vi "writeSerialCommunicator.vi"(8 "error in (no error)":errorcluster, 10 "serialCommunicator":refnum<class "SerialCommunicator.lvclass">, 11 "TEI9150 in":refnum<class "Tovey9150.lvclass">) -> (0 "error out":errorcluster, 3 "TEI9150 out":refnum<class "Tovey9150.lvclass">)   [LabVIEW 2015]
uses:
  Tovey9150.lvclass
  <userlib>/Common/SerialProtocols/SerialCommunicator/SerialCommunicator.lvclass
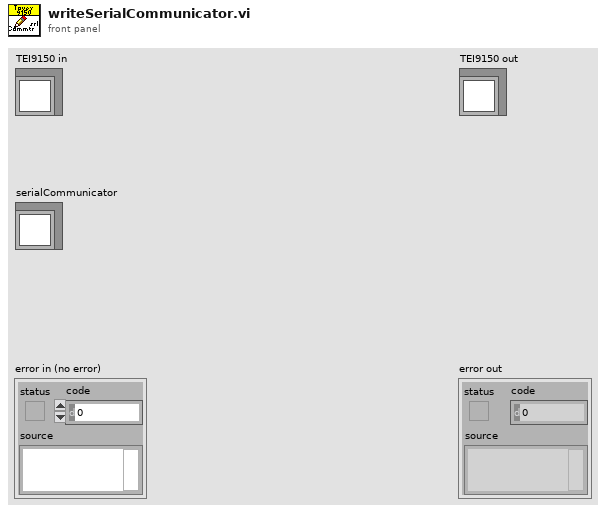
[diagram p1: front panel]
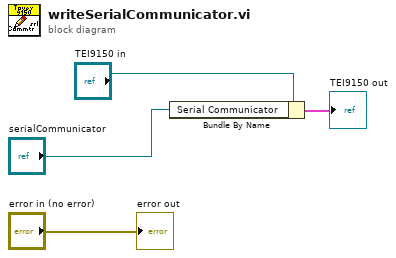
[diagram p0: block diagram]
diagram:
  n1 = Bundle By Name(cluster="TEI9150 in", "Serial Communicator"="serialCommunicator") -> (→"TEI9150 out":cluster{})
  "error out" <- "error in (no error)"
